vi "Creat serial number.vi"(8 "error in (no error)":errorcluster) -> (0 "error out":errorcluster, 2 "date/time string":string, 3 "SN":string)   [LabVIEW 2014]
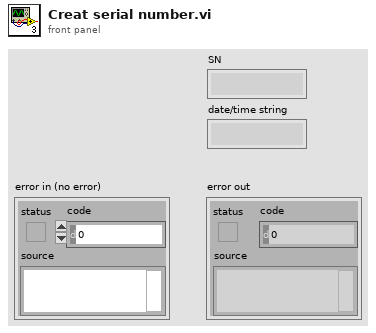
[diagram p1: front panel]
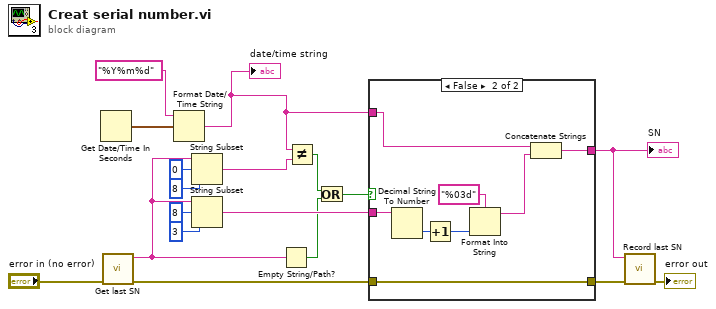
[diagram p0: block diagram]
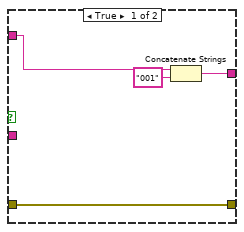
[diagram p2: hidden frame]
diagram:
  n1 = Get Date/Time In Seconds() -> (seconds since 1Jan1904=w18:timestamp)
  n2 = call "Get last SN.vi"("error in (no error)"="error in (no error)") -> ("error out"=w8:errorcluster, "Last SN"=w5:string)  [unwired: 9 in]
  n3 = Format Date/Time String(time format string (%c)="%Y%m%d", seconds (now)=w18) -> (date/time string=w10:string)  [unwired: 1 in]
  "date/time string" <- w10
  n4 = String Subset(string=w5, offset (0)=0, length (rest)=8 ("length (rest)")) -> (substring=w11:string)
  n5 = String Subset(string=w5, offset (0)=8, length (rest)=3 ("length (rest)")) -> (substring=w9:string)
  n6 = Empty String/Path?(string/path=w5) -> (empty?=w3:bool)
  n7 = Not Equal?(x=w10, y=w11) -> (x != y?=w4:bool)
  n8 = Or(x=w4, y=w3) -> (x .or. y?=w2:bool)
  n9 = case shown="False" w2 {
    tunnel: w10 -> [w22 w28]
    tunnel: w9 -> [_ w30]
    tunnel: [w21 w27] -> w6
    tunnel: w8 -> [w19 w26]
    tunnel: [w19 w26] -> w7
    frame True {
      n10 = Concatenate Strings(w22, "001" ("string")) -> (w21:string)
    }
    frame False {
      n11 = Decimal String To Number(string=w30) -> (number=w29:i32)  [unwired: 2 in, 1 out]
      n12 = Increment(x=w29) -> (x+1=w25:i32)
      n13 = Format Into String(format string="%03d", w25) -> (resulting string=w24:string)  [unwired: 2 in, 1 out]
      n14 = Concatenate Strings(w28, w24) -> (w27:string)
    }
  }
  "SN" <- w6
  n15 = call "Record last SN.vi"("error in (no error)"=w7, "Last SN"=w6) -> ("error out"=→"error out":errorcluster)  [unwired: 8 in]
